vi "Set Initialization Data - Analog Signal.vi"(8 "error in":errorcluster, 11 "Head Worker in":refnum<class "Head Worker.lvclass">) -> (0 "error out":errorcluster, 3 "Head Worker out":refnum<class "Head Worker.lvclass">)   [LabVIEW 2023, in "Head Worker.lvclass"]
doc: "In this VI you can set the initialization data of a statically-linked subWorker."
uses:
  Head Worker.lvclass
  Analog Signal/Initialization Data.ctl
  Analog Signal/Response Cases.ctl
  Analog Signal/Support/Signal Type.ctl
  Analog Signal/Support/Signal Config.ctl
  Analog Signal/Support/Sampling Config.ctl
  <vilib>/addons/_Workers/Library/Case Label.ctl
  Head Worker.lvclass/Head Worker.ctl
  Analog Signal/Analog Signal.lvclass
  C:/Program Files (x86)/National Instruments/LabVIEW 2023/vi.lib/addons/_Workers/Library/Classes/Worker/Worker.lvclass
  <vilib>/addons/_Workers/Library/Workers.lvlib
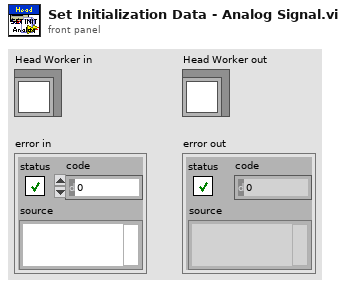
[diagram p1: front panel]
types:
  T1 = typedef "Analog Signal.lvclass/Sampling Config.ctl" = cluster{"Fs":dbl, "#s":dbl}
  T2 = typedef "Analog Signal.lvclass/Signal Config.ctl" = cluster{"offset":dbl, "frequency":dbl, "amplitude":dbl}
  T3 = typedef "Analog Signal.lvclass/Signal Type.ctl" = enum16{"Sine Wave", "Square Wave"}
  T4 = typedef "Analog Signal.lvclass/Initialization Data.ctl" = cluster{"Response Cases":T5}
  T5 = typedef "Analog Signal.lvclass/Response Cases.ctl" = cluster{"Signal Type":T3, "Signal_Config":T2, "Sampling_Config":T1, "Acquisition":T6}
  T6 = typedef "Workers.lvlib/Case Label.ctl" = string
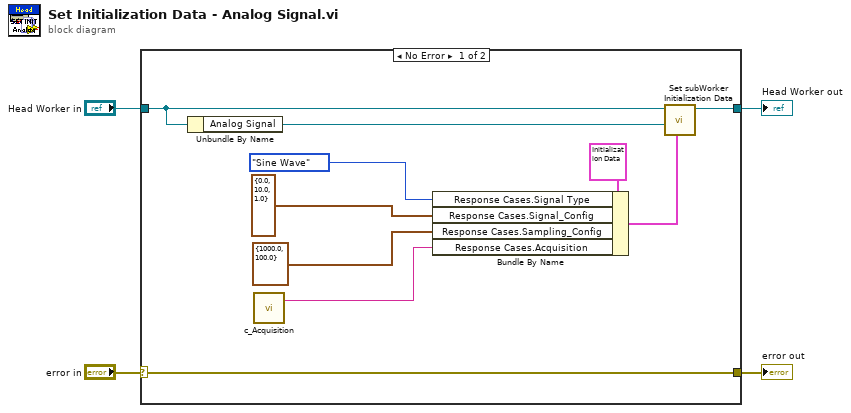
[diagram p0: block diagram]
diagram:
  n1 = case shown="No Error" "error in" {
    selector: "error in" -> [w14 w16]
    tunnel: [w14 w16] -> w3
    tunnel: [w12 w15] -> w2
    tunnel: "Head Worker in" -> [w11 w15]
    frame No Error {
      n2 = Unbundle By Name(w11) -> ("Analog Signal"=w13:refnum<class "Analog Signal.lvclass">)
      n3 = call "c_Acquisition.vi"() -> ("Case Label"=w5:T6)  [unwired: 1 in]
      n4 = Bundle By Name(cluster=T4 {"Response Cases"={"Signal Type"=enum."Sine Wave", "Signal_Config"={"offset"=0.0, "frequency"=10.0, "amplitude"=1.0}, "Sampling_Config"={"Fs"=1000.0, "#s"=1000.0}, "Acquisition"=""}} ("Initialization Data"), "Response Cases.Signal Type"=Signal_Type."Sine Wave", "Response Cases.Signal_Config"=T2 {"offset"=0.0, "frequency"=10.0, "amplitude"=1.0}, "Response Cases.Sampling_Config"=T1 {"Fs"=1000.0, "#s"=100.0}, "Response Cases.Acquisition"=w5) -> (w9:T4)
      n5 = call-dynamic "Set subWorker Initialization Data.vi"("Initialization Data"=w9, "subWorker"=w13, "Worker"=w11) -> ("Worker out"=w12:refnum<class "Head Worker.lvclass">)  [unwired: 8 in]
    }
    frame Error {
    }
  }
  "error out" <- w3
  "Head Worker out" <- w2
